vi "Wait2.0.vi"(10 "Seconds":dbl, 11 "Start Time":u32) -> (3 "Output":bool)   [LabVIEW 2017]
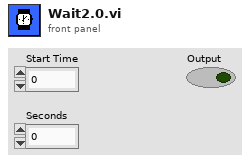
[diagram p1: front panel]
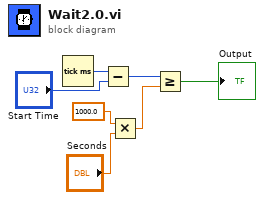
[diagram p0: block diagram]
diagram:
  n1 = Tick Count (ms)() -> (millisecond timer value=w2:u32)
  n2 = Subtract(x=w2, y="Start Time") -> (x-y=w3:u32)
  n3 = Multiply(x=1000.0, y="Seconds") -> (x*y=w4:dbl)
  n4 = Greater Or Equal?(x=w3, y=w4) -> (x >= y?=→"Output":bool)
